vi "Arm Position Indicator Enum.vi"() -> ()   [LabVIEW 2013]
uses:
  Arm State Enum Typedef.ctl
panel:
  in  "Low Goal Button":bool
  in  "Trust Button":bool
  in  "Pick-up Button":bool
  out "Current Arm State":T1(ring)
  in  "Previous Arm State":T1(ring)
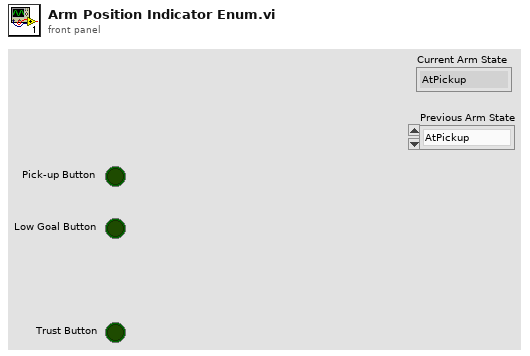
[diagram p1: front panel]
types:
  T1 = enum16{"AtPickup", "MovingDownToPickup", "MovingUpToLowGoal", "AtLowGoal", "MovingDownToLowGoal", "MovingUpToShoot", "AtShoot", "MovingDownToShoot", "MovingUpToTruss", "AtTruss"}
  T2 = typedef "Arm State Enum Typedef.ctl" = enum16{"AtPickup", "MovingDownToPickup", "MovingUpToShoot", "AtShoot", "MovingDownToShoot", "MovingUpToTruss", "AtTruss"}
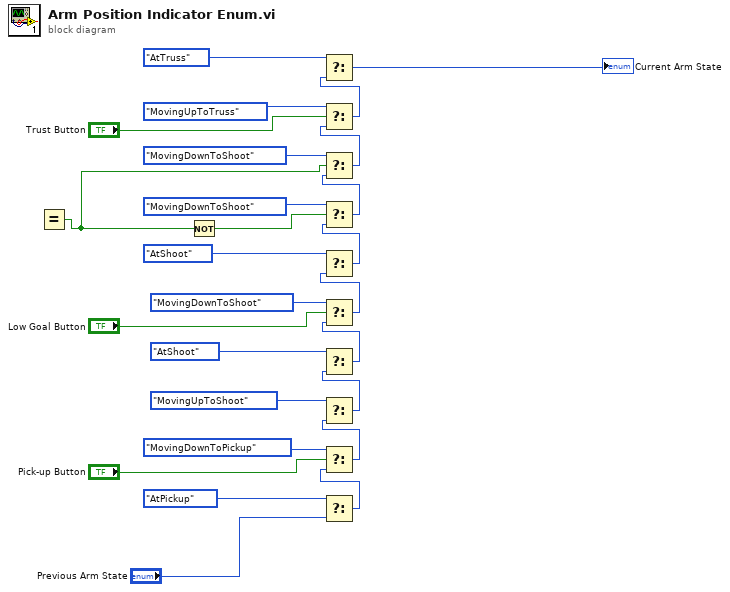
[diagram p0: block diagram]
diagram:
  n1 = Equal?() -> (x = y?=w1:bool)  [unwired: 2 in]
  n2 = Not(x=w1) -> (.not. x?=w2:bool)
  n3 = Select(t=Arm_State_Enum_Typedef."AtPickup" ("Arm State"), f="Previous Arm State") -> (s? t:f=w18:u16)  [unwired: 1 in]
  n4 = Select(t=Arm_State_Enum_Typedef."MovingDownToPickup" ("Arm State"), s="Pick-up Button", f=w18) -> (s? t:f=w19:u16)
  n5 = Select(t=Arm_State_Enum_Typedef."MovingUpToShoot" ("Arm State"), f=w19) -> (s? t:f=w20:u16)  [unwired: 1 in]
  n6 = Select(t=Arm_State_Enum_Typedef."AtShoot" ("Arm State"), f=w20) -> (s? t:f=w21:u16)  [unwired: 1 in]
  n7 = Select(t=Arm_State_Enum_Typedef."MovingDownToShoot" ("Arm State"), s="Low Goal Button", f=w21) -> (s? t:f=w22:u16)
  n8 = Select(t=Arm_State_Enum_Typedef."AtShoot" ("Arm State"), f=w22) -> (s? t:f=w23:u16)  [unwired: 1 in]
  n9 = Select(t=Arm_State_Enum_Typedef."MovingDownToShoot" ("Arm State"), s=w2, f=w23) -> (s? t:f=w24:u16)
  n10 = Select(t=Arm_State_Enum_Typedef."MovingDownToShoot" ("Arm State"), s=w1, f=w24) -> (s? t:f=w25:u16)
  n11 = Select(t=Arm_State_Enum_Typedef."MovingUpToTruss" ("Arm State"), s="Trust Button", f=w25) -> (s? t:f=w26:u16)
  n12 = Select(t=Arm_State_Enum_Typedef."AtTruss" ("Arm State"), f=w26) -> (s? t:f=→"Current Arm State":u16)  [unwired: 1 in]
